vi "Build Word Initial Raw Values for All Labels.vi"(8 "error in":errorcluster, 11 "Tx Scheduled Labels Execution Unit in":refnum<class "Tx Scheduled Labels Execution Unit.lvclass">) -> (0 "error out":errorcluster, 3 "Tx Scheduled Labels Execution Unit out":refnum<class "Tx Scheduled Labels Execution Unit.lvclass">)   [LabVIEW 2020, in "AIM ARINC 429 Engine.lvlib" / "Implementation.lvlib" / "Tx Scheduled Labels Execution Unit.lvclass"]
uses:
  Tx Scheduled Labels Execution Unit.lvclass
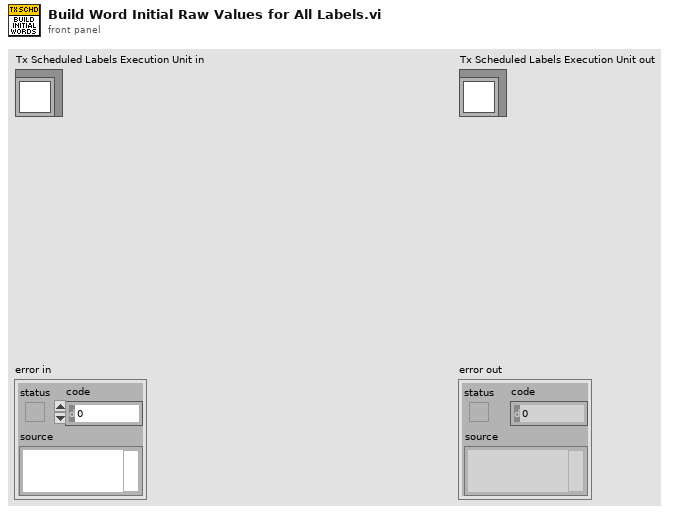
[diagram p1: front panel]
types:
  T1 = typedef "RT Hardware Channel Settings.ctl" = cluster{"channel #":u16, "channel handle":u64, "labels settings for RT":T2[]}
  T2 = typedef "RT Label Settings.ctl" = cluster{"Name":string, "xmlName":string, "label":T3, "transfer period":u32, "SDI_Enabled":bool, "SDI":u8, "parameter driver data":T4, "transfer type":T8, "has timestamp?":bool, "Label Disable/Trigger Channel Reference":T7, "Message Handle":u64, "Initialized?":bool, "Word Initial Raw Value":u32, "Label Timestamp Channel Data Reference":T9, "disabled":bool}
  T3 = typedef "Label.ctl" = u8
  T4 = typedef "RT Parameters.ctl" = cluster{"parameter definitions":T5[], "Tx parameter refs":T7[]}
  T5 = typedef "Parameter Definition.ctl" = cluster{"start index":i32, "size":i32, "encoding":T6, "signed":bool, "scale multiplier":dbl, "scale offset":dbl, "default value":dbl}
  T6 = typedef "Encoding and Decoding.lvlib/Encoding.ctl" = enum16{"BNR", "BCD", "Discrete"}
  T7 = typedef "Custom Device API.lvlib/Custom Device Item Ref.ctl" = u64
  T8 = typedef "Transfer Type.ctl" = enum16{"Scheduled", "Acyclic", "Block", "Strobe"}
  T9 = typedef "Custom Device API.lvlib/Data Reference.ctl" = i32
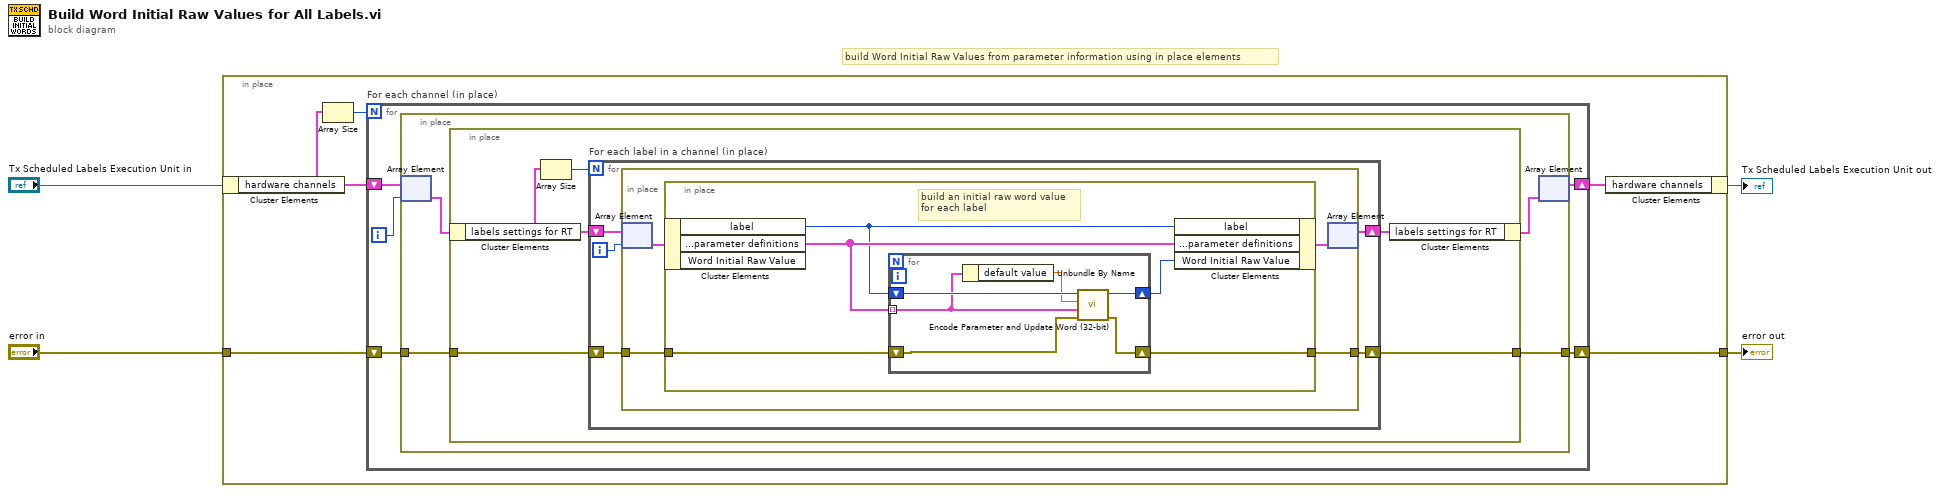
[diagram p0: block diagram]
diagram:
  # "build Word Initial Raw Values from parameter information using in place elements"
  n1 = in-place {
    in-place-border: "error in" -> [w6]
    in-place-border: [w5] -> w1
    n2 = in-place-cluster #1("Tx Scheduled Labels Execution Unit in") -> ("hardware channels"=w7:T1[])
    n3 = Array Size(array=w7) -> (size(s)=w8:i32)
    n4 = for "For each channel (in place)" {
      N: w8 -> [_]
      shift-right: [w12] -> w9
      shift-left: w7 -> [w14]
      shift-right: [w10] -> w5
      shift-left: w6 -> [w11]
      i -> [w13]
      n5 = in-place {
        in-place-border: w11 -> [w16]
        in-place-border: [w15] -> w10
        n6 = in-place-array #2(w14, w13) -> (w18:T1)
        n7 = in-place {
          in-place-border: w16 -> [w20]
          in-place-border: [w19] -> w15
          n8 = in-place-cluster #3(w18) -> ("labels settings for RT"=w22:T2[])
          n9 = Array Size(array=w22) -> (size(s)=w23:i32)
          n10 = for "For each label in a channel (in place)" {
            N: w23 -> [_]
            shift-right: [w26] -> w21
            shift-left: w22 -> [w28]
            shift-right: [w24] -> w19
            shift-left: w20 -> [w25]
            i -> [w27]
            n11 = in-place {
              in-place-border: w25 -> [w30]
              in-place-border: [w29] -> w24
              n12 = in-place-array #4(w28, w27) -> (w32:T2)
              n13 = in-place {
                in-place-border: w30 -> [w36]
                in-place-border: [w35] -> w29
                # "build an initial raw word value\nfor each label"
                n14 = in-place-cluster #5(w32) -> ("label"=w34:T3, "parameter driver data.parameter definitions"=w37:T5[])  [unwired: 1 out]
                n15 = for {
                  shift-right: [w42] -> w33
                  shift-left: w34 -> [w43]
                  tunnel: w37 -> [w38] mode=indexing
                  shift-right: [w41] -> w35
                  shift-left: w36 -> [w39]
                  n16 = Unbundle By Name(w38) -> ("default value"=w40:dbl)
                  n17 = call "Encode Parameter and Update Word (32-bit).vi"("error in"=w39, "parameter definition"=w38, "parameter value"=w40, "word in"=w43) -> ("error out"=w41:errorcluster, "word out"=w42:u32)  [unwired: 6 in]
                }
                n18 = in-place-cluster #5("label"=w34, "parameter driver data.parameter definitions"=w37, "Word Initial Raw Value"=w33) -> (w31:T2)
              }
              n19 = in-place-array #4(w31) -> (w26:T2[])  [unwired: 1 out]
            }
          }
          n20 = in-place-cluster #3("labels settings for RT"=w21) -> (w17:T1)
        }
        n21 = in-place-array #2(w17) -> (w12:T1[])  [unwired: 1 out]
      }
    }
    n22 = in-place-cluster #1("hardware channels"=w9) -> (→"Tx Scheduled Labels Execution Unit out":refnum<class "Tx Scheduled Labels Execution Unit.lvclass">)
  }
  "error out" <- w1
